vi "testReadData.vi"() -> ()   [LabVIEW 2025]
panel:
  out "error out":errorcluster
  out "Waveform Chart 2":u8[](graph)
  in  "Start":bool
  in  "stop":bool
  in  "Horizontal Slide Switch":bool
  out "error out 2":errorcluster
  out "read buffer":string
  in  "VISA resource name":refnum<visa-resource-name>
  out "Waveform Chart":u8[](graph)
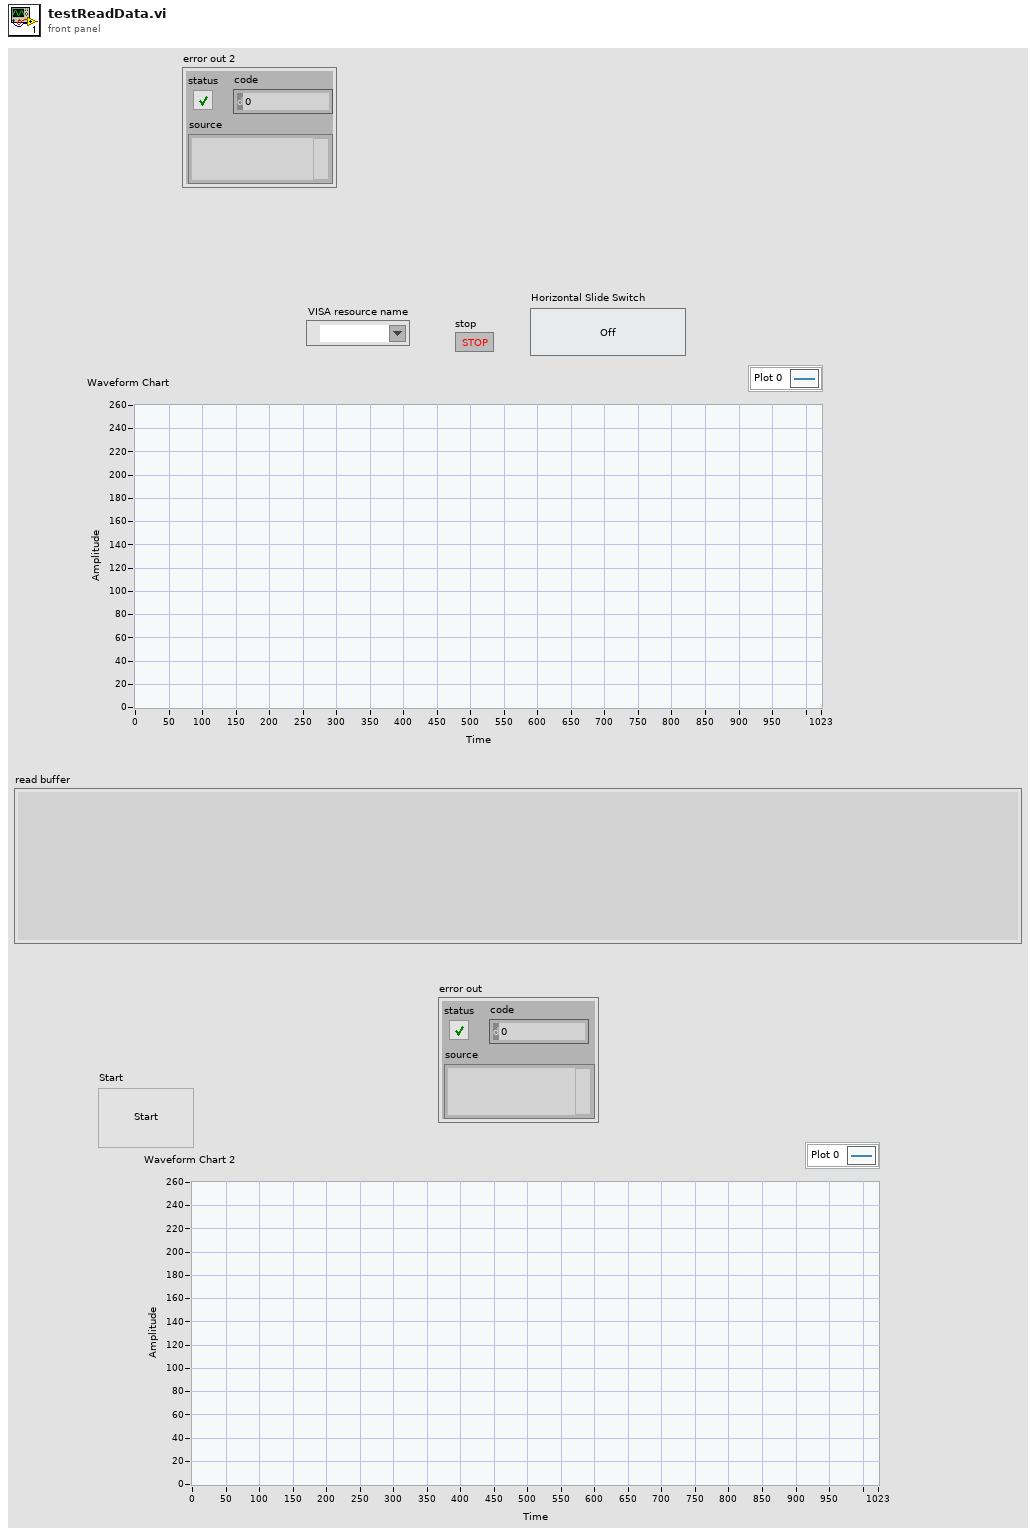
[diagram p1: front panel]
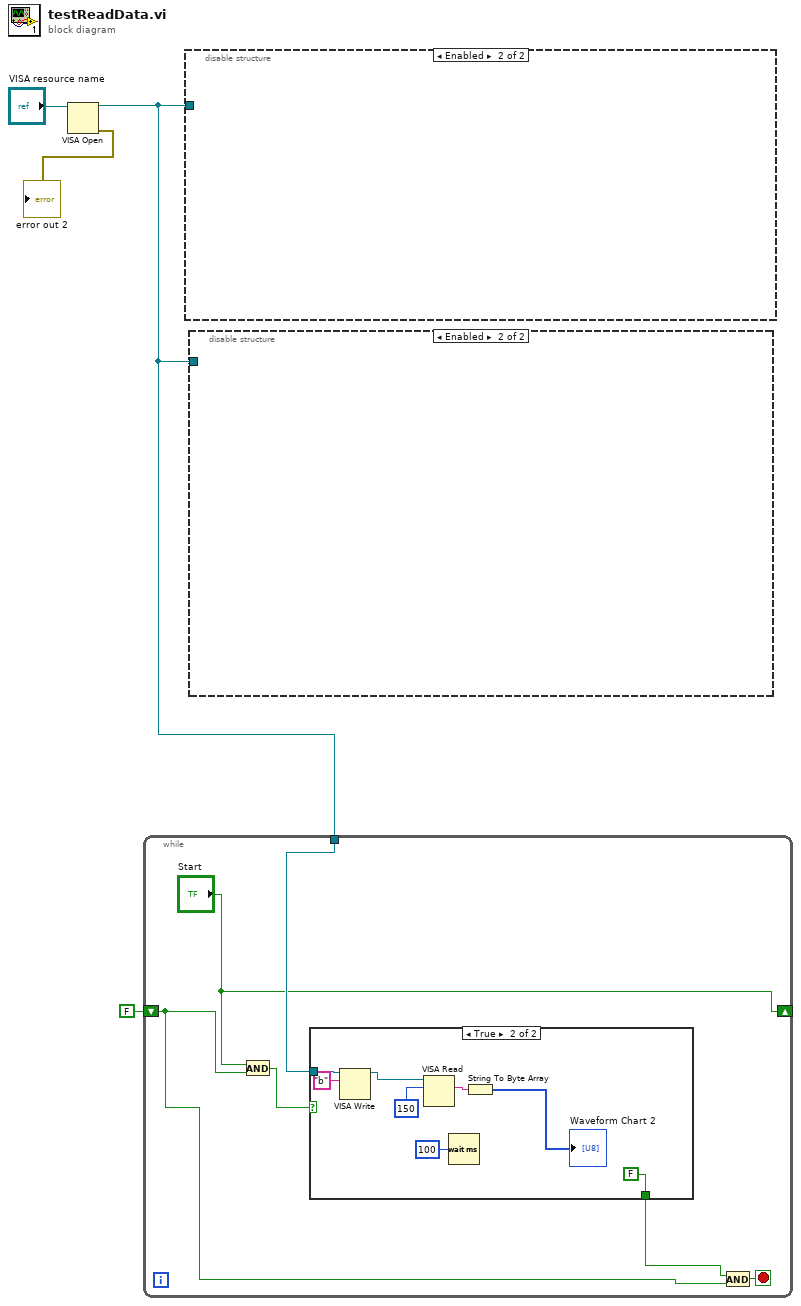
[diagram p0: block diagram]
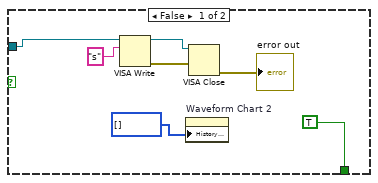
[diagram p2: hidden frame]
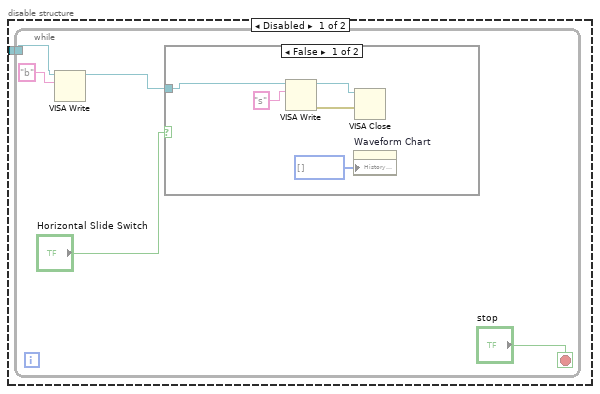
[diagram p3: hidden frame]
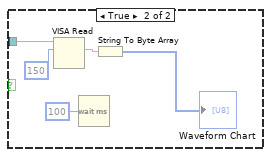
[diagram p4: hidden frame]
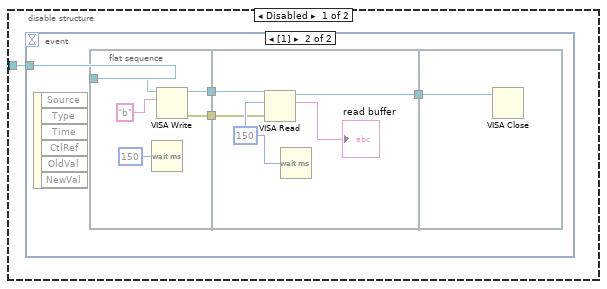
[diagram p5: hidden frame]
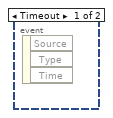
[diagram p6: hidden frame]
diagram:
  n1 = VISA Open(VISA resource name="VISA resource name") -> (VISA resource name=w2:refnum<visa-resource-name>, error out=→"error out 2":errorcluster)  [unwired: 4 in]
  n2 = while {
    tunnel: w2 -> [w10]
    shift-right: ["Start"] -> _
    shift-left: FALSE -> [w5]
    stop <- w9 stop-if-true
    n3 = And(x="Start", y=w5) -> (x .and. y?=w7:bool)
    n4 = case shown="True" w7 {
      tunnel: w10 -> [w14 w19]
      tunnel: [TRUE FALSE] -> w8
      frame False {
        n5 = VISA Write(VISA resource name=w14, write buffer="s") -> (VISA resource name out=w16:refnum<visa-resource-name>, error out=w17:errorcluster)  [unwired: 1 in, 1 out]
        n6 = property on="Waveform Chart 2" class="WFChart (strict)"("History Data"=u8[] [] ("Waveform Chart 2")) -> ()  [unwired: 2 in, 2 out]
        n7 = VISA Close(VISA resource name=w16, error in (no error)=w17) -> (error out=→"error out":errorcluster)
      }
      frame True {
        n8 = VISA Write(VISA resource name=w19, write buffer="b") -> (VISA resource name out=w25:refnum<visa-resource-name>)  [unwired: 1 in, 2 out]
        n9 = VISA Read(VISA resource name=w25, byte count=u32 150) -> (read buffer=w23:string)  [unwired: 1 in, 3 out]
        n10 = Wait (ms)(milliseconds to wait=u32 100) -> ()  [unwired: 1 out]
        n11 = String To Byte Array(string=w23) -> (unsigned byte array=→"Waveform Chart 2":u8[])
      }
    }
    n12 = And(x=w8, y=w5) -> (x .and. y?=w9:bool)
  }
  n13 = disable-structure shown="Enabled" {
    disable-tunnel: w2 -> [w26 _]
    frame Disabled {
      n14 = event shown="[1]" {
        selector: _ -> [_ _]
        dyn-events: _ -> [_ _]
        timeout: _ -> [_ _]
        tunnel: w26 -> [_ w30]
        event Timeout {
          n15 = event-data() -> ()  [unwired: 1 in, 3 out]
        }
        event #1 (no event record) {
          n16 = event-data() -> ()  [unwired: 1 in, 6 out]
          n17 = flat-sequence {
            tunnel: w30 -> [w35]
            tunnel: [w32] -> w29
            tunnel: [w31] -> w28
            tunnel: w29 -> [w38]
            tunnel: w28 -> [w37]
            tunnel: [w36] -> w27
            tunnel: w27 -> [w41]
            frame #0 {
              n18 = Wait (ms)(milliseconds to wait=u32 150) -> ()  [unwired: 1 out]
              n19 = VISA Write(VISA resource name=w35, write buffer="b") -> (VISA resource name out=w32:refnum<visa-resource-name>, error out=w31:errorcluster)  [unwired: 1 in, 1 out]
            }
            frame #1 {
              w39 = u32 150 ("byte count")
              n20 = VISA Read(VISA resource name=w38, byte count=w39, error in (no error)=w37) -> (VISA resource name out=w36:refnum<visa-resource-name>, read buffer=→"read buffer":string)  [unwired: 2 out]
              n21 = Wait (ms)(milliseconds to wait=w39) -> ()  [unwired: 1 out]
            }
            frame #2 {
              n22 = VISA Close(VISA resource name=w41) -> ()  [unwired: 1 in, 1 out]
            }
          }
        }
      }
    }
    frame Enabled {
    }
  }
  n23 = disable-structure shown="Enabled" {
    disable-tunnel: w2 -> [w42 _]
    frame Disabled {
      n24 = while {
        tunnel: w42 -> [w46]
        stop <- "stop" stop-if-true
        n25 = VISA Write(VISA resource name=w46, write buffer="b") -> (VISA resource name out=w45:refnum<visa-resource-name>)  [unwired: 1 in, 2 out]
        n26 = case shown="False" "Horizontal Slide Switch" {
          tunnel: w45 -> [w48 w54]
          frame False {
            n27 = VISA Write(VISA resource name=w48, write buffer="s") -> (VISA resource name out=w52:refnum<visa-resource-name>, error out=w51:errorcluster)  [unwired: 1 in, 1 out]
            n28 = property on="Waveform Chart" class="WFChart (strict)"("History Data"=u8[] []) -> ()  [unwired: 2 in, 2 out]
            n29 = VISA Close(VISA resource name=w52, error in (no error)=w51) -> ()  [unwired: 1 out]
          }
          frame True {
            n30 = VISA Read(VISA resource name=w54, byte count=u32 150) -> (read buffer=w56:string)  [unwired: 1 in, 3 out]
            n31 = Wait (ms)(milliseconds to wait=u32 100) -> ()  [unwired: 1 out]
            n32 = String To Byte Array(string=w56) -> (unsigned byte array=→"Waveform Chart":u8[])
          }
        }
      }
    }
    frame Enabled {
    }
  }
